vi "init servo.vi"(11 "VISA引用句柄输入":refnum<visa-resource-name>) -> (0 "错误输出":errorcluster, 3 "Arduino Resource":T1)   [LabVIEW 2016]
uses:
  <vilib>/LabVIEW Interface for Arduino/Type Defs/Arduino Resource.ctl
  <vilib>/LabVIEW Interface for Arduino/Type Defs/Board Type.ctl
  <vilib>/LabVIEW Interface for Arduino/LabVIEW Interface for Arduino.lvlib
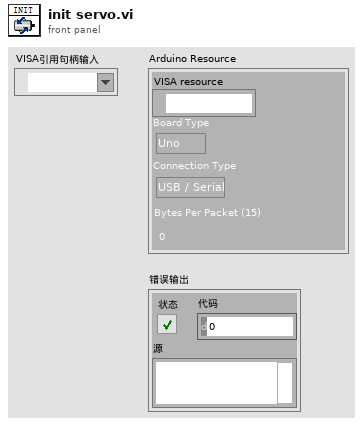
[diagram p1: front panel]
types:
  T1 = typedef "LabVIEW Interface for Arduino.lvlib/Arduino Resource.ctl" = cluster{"VISA resource":refnum<visa-resource-name>, "Board Type":T2, "Connection Type":enum8{"USB / Serial"}, "Bytes Per Packet (15)":u8}
  T2 = typedef "LabVIEW Interface for Arduino.lvlib/Board Type.ctl" = enum16{"Uno", "Dimuelanove w/Atmega 328", "Mega 2560"}
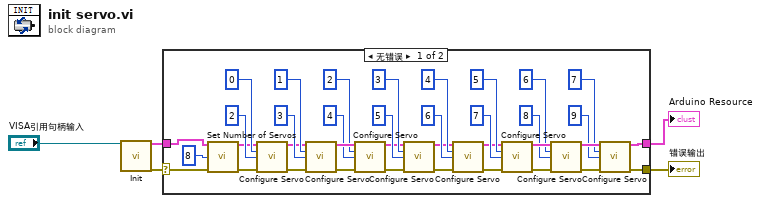
[diagram p0: block diagram]
diagram:
  n1 = call <vilib>:"Init.vi"("VISA resource"="VISA引用句柄输入") -> ("Arduino Resource"=w2:T1, "error out"=w1:errorcluster)  [unwired: 17 in]
  n2 = case shown="无错误" w1 {
    selector: w1 -> [w16 w43]
    tunnel: [w6 w43] -> w5
    tunnel: [w7 w44] -> w4
    tunnel: w2 -> [w17 w44]
    frame No Error {
      n3 = call <vilib>:"Set Number of Servos.vi"("Arduino Resource"=w17, "Number Of Servos (1)"=u8 8 ("Number of Servos"), "error in"=w16) -> ("Arduino Resource"=w19:T1, "error out"=w20:errorcluster)  [unwired: 11 in]
      n4 = call <vilib>:"Configure Servo.vi"("Arduino Resource"=w19, "Servo Number (0)"=u8 0 ("Servo Number"), "DIO Pin (2)"=u8 2 ("Servo Number"), "error in"=w20) -> ("Arduino Resource"=w21:T1, "error out"=w35:errorcluster)  [unwired: 10 in]
      n5 = call <vilib>:"Configure Servo.vi"("Arduino Resource"=w21, "Servo Number (0)"=u8 1 ("Servo Number"), "DIO Pin (2)"=u8 3 ("Servo Number"), "error in"=w35) -> ("Arduino Resource"=w34:T1, "error out"=w36:errorcluster)  [unwired: 10 in]
      n6 = call <vilib>:"Configure Servo.vi"("Arduino Resource"=w34, "Servo Number (0)"=u8 2, "DIO Pin (2)"=u8 4, "error in"=w36) -> ("Arduino Resource"=w26:T1, "error out"=w37:errorcluster)  [unwired: 10 in]
      n7 = call <vilib>:"Configure Servo.vi"("Arduino Resource"=w26, "Servo Number (0)"=u8 3, "DIO Pin (2)"=u8 5, "error in"=w37) -> ("Arduino Resource"=w31:T1, "error out"=w38:errorcluster)  [unwired: 10 in]
      n8 = call <vilib>:"Configure Servo.vi"("Arduino Resource"=w31, "Servo Number (0)"=u8 4, "DIO Pin (2)"=u8 6, "error in"=w38) -> ("Arduino Resource"=w39:T1, "error out"=w40:errorcluster)  [unwired: 10 in]
      n9 = call <vilib>:"Configure Servo.vi"("Arduino Resource"=w39, "Servo Number (0)"=u8 5, "DIO Pin (2)"=u8 7, "error in"=w40) -> ("Arduino Resource"=w15:T1, "error out"=w14:errorcluster)  [unwired: 10 in]
      n10 = call <vilib>:"Configure Servo.vi"("Arduino Resource"=w15, "Servo Number (0)"=u8 6, "DIO Pin (2)"=u8 8, "error in"=w14) -> ("Arduino Resource"=w11:T1, "error out"=w10:errorcluster)  [unwired: 10 in]
      n11 = call <vilib>:"Configure Servo.vi"("Arduino Resource"=w11, "Servo Number (0)"=u8 7, "DIO Pin (2)"=u8 9, "error in"=w10) -> ("Arduino Resource"=w7:T1, "error out"=w6:errorcluster)  [unwired: 10 in]
    }
    frame Error {
    }
  }
  "错误输出" <- w5
  "Arduino Resource" <- w4
